vi "Close.vi"(8 "error in (no error)":errorcluster, 11 "Data in":refnum<class "Abs_I64 Integer.lvclass">) -> (0 "error out":errorcluster, 3 "Data out":refnum<class "Abs_I64 Integer.lvclass">)   [LabVIEW 2021, in "Abs_I64 Integer.lvclass"]
uses:
  Abs_I64 Integer.lvclass
  Integer/Abs_Integer.lvclass
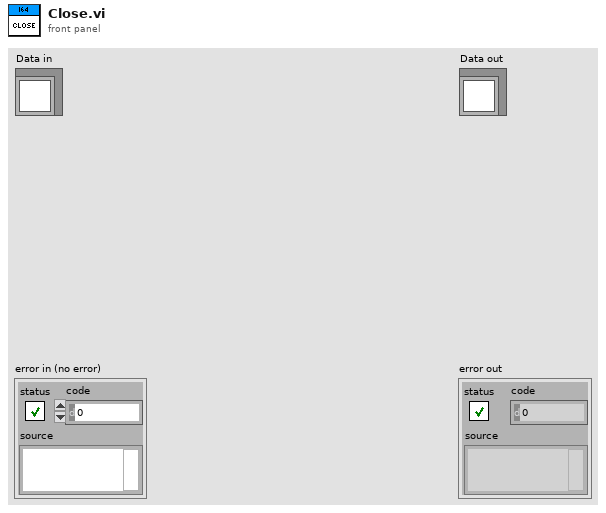
[diagram p1: front panel]
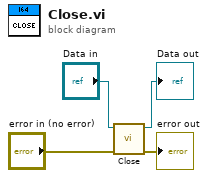
[diagram p0: block diagram]
diagram:
  n1 = call-parent "Close.vi"("error in (no error)"="error in (no error)", "Data in"="Data in") -> ("error out"=→"error out":errorcluster, "Data out"=→"Data out":refnum<class "Abs_I64 Integer.lvclass">)  [unwired: 8 in]
